vi "Player Name.vi"(11 "MyTeam in":refnum<class "MyTeam.lvclass">) -> (2 "Player Name":string)   [LabVIEW 2020, in "Galaxy.lvlib" / "MyTeam.lvclass"]
uses:
  MyTeam.lvclass
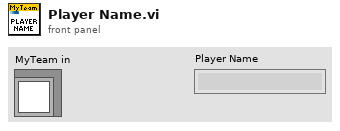
[diagram p1: front panel]
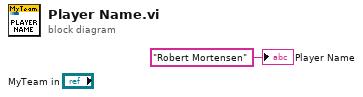
[diagram p0: block diagram]
diagram:
  "Player Name" <- "Robert Mortensen" ("Player Name")
